vi "Plaintext CW Map Creator.vi"() -> (3 "Plaintext to CW Map":map{string, bool[]}(c390))   [LabVIEW 2026]
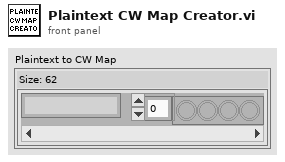
[diagram p1: front panel]
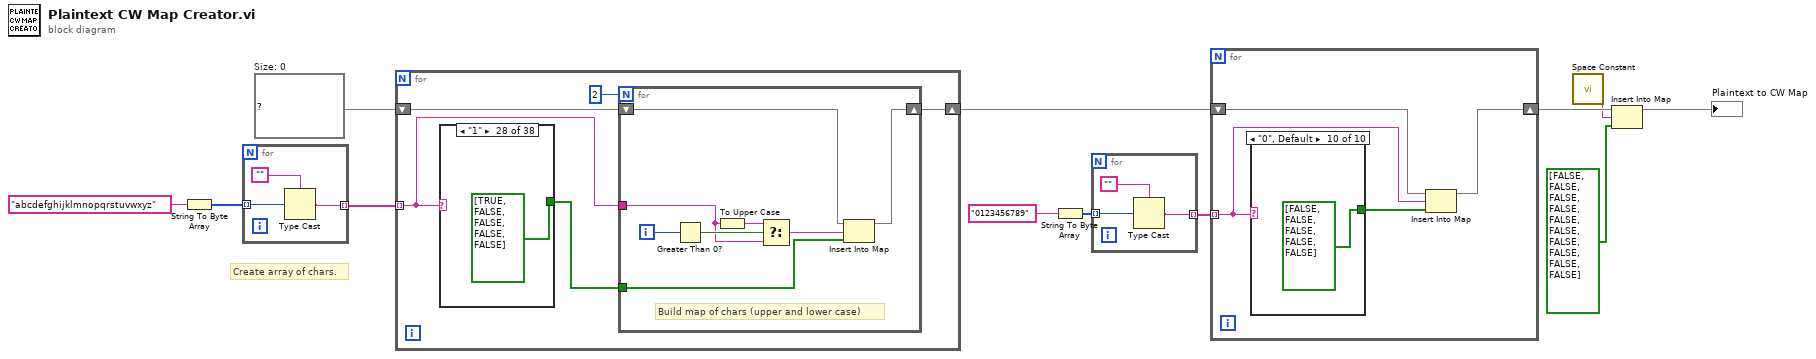
[diagram p0: block diagram]
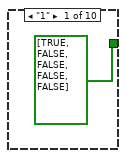
[diagram p2: hidden frame]
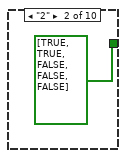
[diagram p3: hidden frame]
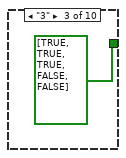
[diagram p4: hidden frame]
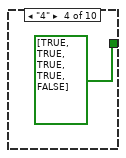
[diagram p5: hidden frame]
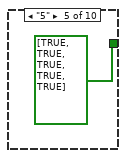
[diagram p6: hidden frame]
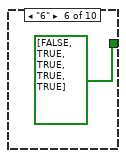
[diagram p7: hidden frame]
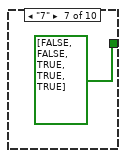
[diagram p8: hidden frame]
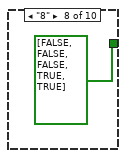
[diagram p9: hidden frame]
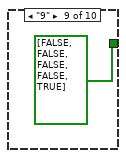
[diagram p10: hidden frame]
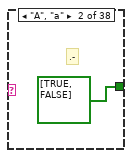
[diagram p12: hidden frame]
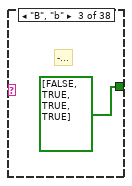
[diagram p13: hidden frame]
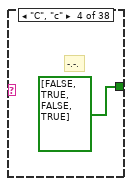
[diagram p14: hidden frame]
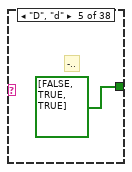
[diagram p15: hidden frame]
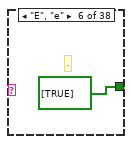
[diagram p16: hidden frame]
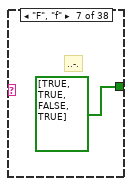
[diagram p17: hidden frame]
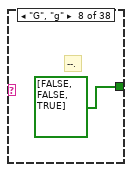
[diagram p18: hidden frame]
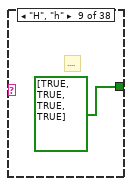
[diagram p19: hidden frame]
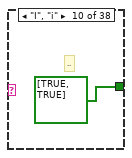
[diagram p20: hidden frame]
diagram:
  w9 = map{string, bool[]} {}  # Size: 0
  # "Create array of chars."
  n1 = String To Byte Array(string="abcdefghijklmnopqrstuvwxyz") -> (unsigned byte array=w11:u8[])
  n2 = for {
    tunnel: w11 -> [w15] mode=indexing
    tunnel: [w13] -> w10 mode=indexing
    n3 = Type Cast(type="", x=w15) -> (*(type *) &x=w13:string)
  }
  n4 = for {
    tunnel: w10 -> [w16] mode=indexing
    shift-right: [w18] -> w5
    shift-left: w9 -> [w19]
    n5 = case shown="\"1\"" w16 {
      tunnel: [_ bool[] [TRUE, FALSE] bool[] [FALSE, TRUE, TRUE, TRUE] bool[] [FALSE, TRUE, FALSE, TRUE] bool[] [FALSE, TRUE, TRUE] bool[] [TRUE] bool[] [TRUE, TRUE, FALSE, TRUE] bool[] [FALSE, FALSE, TRUE] bool[] [TRUE, TRUE, TRUE, TRUE] bool[] [TRUE, TRUE] bool[] [TRUE, FALSE, FALSE, FALSE] bool[] [FALSE, TRUE, FALSE] bool[] [TRUE, FALSE, TRUE, TRUE] bool[] [FALSE, FALSE] bool[] [FALSE, TRUE] bool[] [FALSE, FALSE, FALSE] bool[] [TRUE, FALSE, FALSE, TRUE] bool[] [FALSE, FALSE, TRUE, FALSE] bool[] [TRUE, FALSE, TRUE] bool[] [TRUE, TRUE, TRUE] bool[] [FALSE] bool[] [TRUE, TRUE, FALSE] bool[] [TRUE, TRUE, TRUE, FALSE] bool[] [TRUE, FALSE, FALSE] bool[] [FALSE, TRUE, TRUE, FALSE] bool[] [FALSE, TRUE, FALSE, FALSE] bool[] [FALSE, FALSE, TRUE, TRUE] bool[] [TRUE, FALSE, FALSE, FALSE, FALSE] bool[] [TRUE, TRUE, FALSE, FALSE, FALSE] bool[] [TRUE, TRUE, TRUE, FALSE, FALSE] bool[] [TRUE, TRUE, TRUE, TRUE, FALSE] bool[] [TRUE, TRUE, TRUE, TRUE, TRUE] bool[] [FALSE, TRUE, TRUE, TRUE, TRUE] bool[] [FALSE, FALSE, TRUE, TRUE, TRUE] bool[] [FALSE, FALSE, FALSE, TRUE, TRUE] bool[] [FALSE, FALSE, FALSE, FALSE, TRUE] bool[] [FALSE, FALSE, FALSE, FALSE, FALSE] bool[] [TRUE, TRUE, FALSE, FALSE, TRUE, TRUE]] -> w17
      frame "", Default {
      }
      frame "A", "a" {
        # ".-"
      }
      frame "B", "b" {
        # "-..."
      }
      frame "C", "c" {
        # "-.-."
      }
      frame "D", "d" {
        # "-.."
      }
      frame "E", "e" {
        # "."
      }
      frame "F", "f" {
        # "..-."
      }
      frame "G", "g" {
        # "--."
      }
      frame "H", "h" {
        # "...."
      }
      frame "I", "i" {
        # ".."
      }
      frame "J", "j" {
        # ".---"
      }
      frame "K", "k" {
        # "-.-"
      }
      frame "L", "l" {
        # ".-.."
      }
      frame "M", "m" {
        # "--"
      }
      frame "N", "n" {
        # "-."
      }
      frame "O", "o" {
        # "---"
      }
      frame "P", "p" {
        # ".--."
      }
      frame "Q", "q" {
        # "--.-"
      }
      frame "R", "r" {
        # ".-."
      }
      frame "S", "s" {
        # "..."
      }
      frame "T", "t" {
        # "-"
      }
      frame "U", "u" {
        # "..-"
      }
      frame "V", "v" {
        # "...-"
      }
      frame "W", "w" {
        # ".--"
      }
      frame "X", "x" {
        # "-..-"
      }
      frame "Y", "y" {
        # "-.--"
      }
      frame "Z", "z" {
        # "--.."
      }
      frame "1" {
      }
      frame "2" {
      }
      frame "3" {
      }
      frame "4" {
      }
      frame "5" {
      }
      frame "6" {
      }
      frame "7" {
      }
      frame "8" {
      }
      frame "9" {
      }
      frame "0" {
      }
      frame "?" {
        # "..--.."
      }
    }
    n6 = for {
      N: 2 -> [_]
      tunnel: w16 -> [w62]
      shift-right: [w59] -> w18
      shift-left: w19 -> [w60]
      tunnel: w17 -> [w58]
      i -> [w65]
      # "Build map of chars (upper and lower case)"
      n7 = Greater Than 0?(x=w65) -> (x > 0?=w64:bool)
      n8 = To Upper Case(1:w62) -> (0:w63:string)
      n9 = Select(t=w63, s=w64, f=w62) -> (s? t:f=w61:string)
      n10 = Insert Into Map(map in=w60, key=w61, value=w58) -> (map out=w59:map{string, bool[]})  [unwired: 2 out]
    }
  }
  n11 = String To Byte Array(string="0123456789") -> (unsigned byte array=w8:u8[])
  n12 = for {
    tunnel: w8 -> [w68] mode=indexing
    tunnel: [w66] -> w7 mode=indexing
    n13 = Type Cast(type="", x=w68) -> (*(type *) &x=w66:string)
  }
  n14 = for {
    tunnel: w7 -> [w69] mode=indexing
    shift-right: [w70] -> w4
    shift-left: w5 -> [w71]
    n15 = case shown="\"0\", Default" w69 {
      tunnel: [bool[] [TRUE, FALSE, FALSE, FALSE, FALSE] bool[] [TRUE, TRUE, FALSE, FALSE, FALSE] bool[] [TRUE, TRUE, TRUE, FALSE, FALSE] bool[] [TRUE, TRUE, TRUE, TRUE, FALSE] bool[] [TRUE, TRUE, TRUE, TRUE, TRUE] bool[] [FALSE, TRUE, TRUE, TRUE, TRUE] bool[] [FALSE, FALSE, TRUE, TRUE, TRUE] bool[] [FALSE, FALSE, FALSE, TRUE, TRUE] bool[] [FALSE, FALSE, FALSE, FALSE, TRUE] bool[] [FALSE, FALSE, FALSE, FALSE, FALSE]] -> w72
      frame "1" {
      }
      frame "2" {
      }
      frame "3" {
      }
      frame "4" {
      }
      frame "5" {
      }
      frame "6" {
      }
      frame "7" {
      }
      frame "8" {
      }
      frame "9" {
      }
      frame "0", Default {
      }
    }
    n16 = Insert Into Map(map in=w71, key=w69, value=w72) -> (map out=w70:map{string, bool[]})  [unwired: 2 out]
  }
  n17 = call <vilib>:"Space Constant.vi"() -> ("String"=w2:string)
  n18 = Insert Into Map(map in=w4, key=w2, value=bool[] [FALSE, FALSE, FALSE, FALSE, FALSE, FALSE, FALSE, FALSE, FALSE, FALSE]) -> (map out=→"Plaintext to CW Map":map{string, bool[]})  [unwired: 2 out]
